vi "toCluster.vi"(3 "error in (no error)":errorcluster, 5 "PulseData in":refnum<class "PulseData.lvclass">) -> (0 "error out":errorcluster, 1 "Pulse Data Cluster":T1, 2 "PulseData out":refnum<class "PulseData.lvclass">)   [LabVIEW 2013, in "Controls Log Monitor.lvlib" / "PulseData.lvclass"]
uses:
  PulseData.lvclass
  PulseData.lvclass/PulseData.ctl
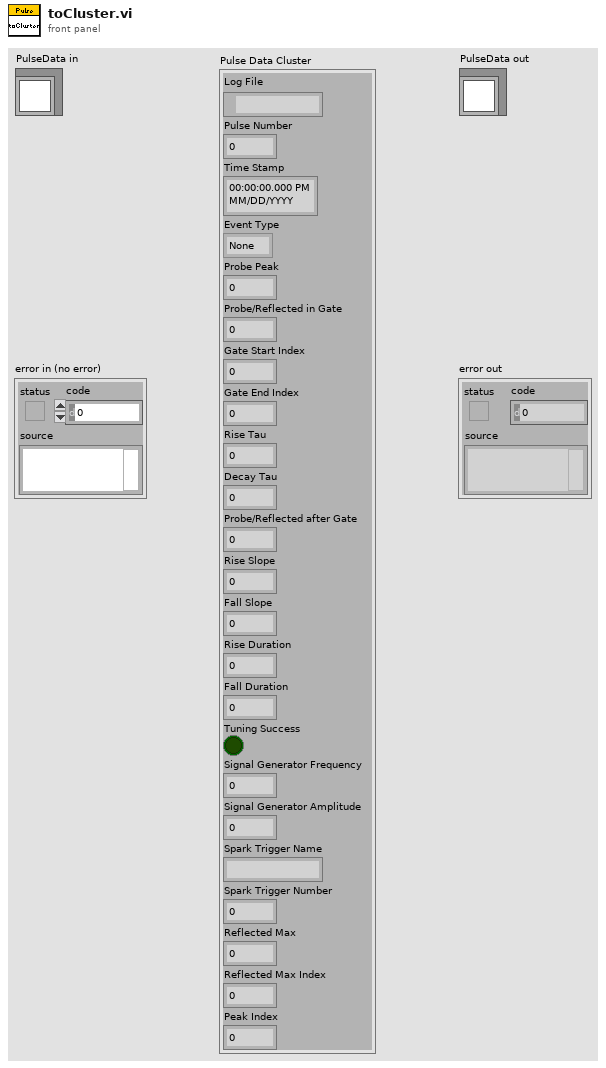
[diagram p1: front panel]
types:
  T1 = cluster{"Log File":path, "Pulse Number":u32, "Time Stamp":timestamp, "Event Type":enum16{"None", "Tune", "Periodic Capture", "Spark Trigger"}, "Probe Peak":dbl, "Probe/Reflected in Gate":dbl, "Gate Start Index":i32, "Gate End Index":i32, "Rise Tau":dbl, "Decay Tau":dbl, "Probe/Reflected after Gate":dbl, "Rise Slope":dbl, "Fall Slope":dbl, "Rise Duration":dbl, "Fall Duration":dbl, "Tuning Success":bool, "Signal Generator Frequency":dbl, "Signal Generator Amplitude":dbl, "Spark Trigger Name":string, "Spark Trigger Number":i32, "Reflected Max":dbl, "Reflected Max Index":i32, "Peak Index":i32}
  T2 = enum16{"None", "Tune", "Periodic Capture", "Spark Trigger"}
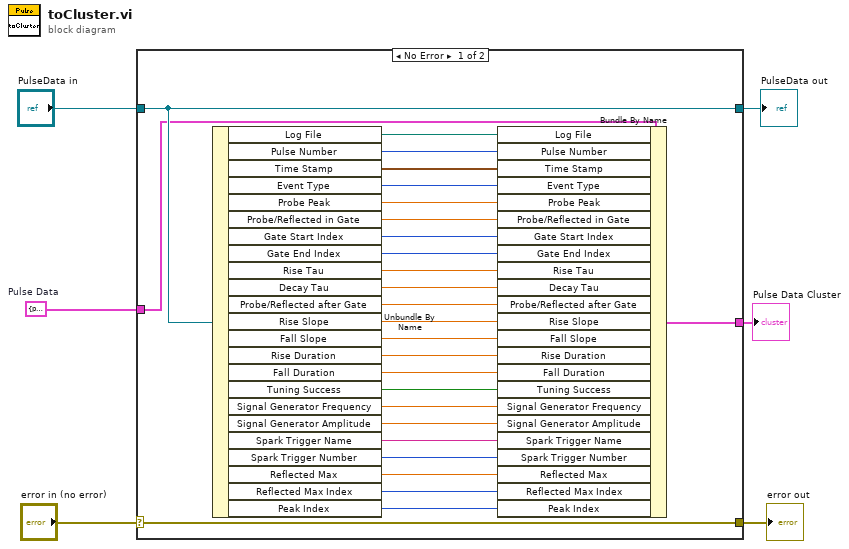
[diagram p0: block diagram]
diagram:
  w2 = T1 {"Log File"=path "", "Pulse Number"=0, "Time Stamp"=timestamp(0 s since 1904-01-01), "Event Type"=enum."None", "Probe Peak"=0.0, "Probe/Reflected in Gate"=0.0, "Gate Start Index"=0, "Gate End Index"=0, "Rise Tau"=0.0, "Decay Tau"=0.0, "Probe/Reflected after Gate"=0.0, "Rise Slope"=0.0, "Fall Slope"=0.0, "Rise Duration"=0.0, "Fall Duration"=0.0, "Tuning Success"=FALSE, "Signal Generator Frequency"=0.0, "Signal Generator Amplitude"=0.0, "Spark Trigger Name"="", "Spark Trigger Number"=0, "Reflected Max"=0.0, "Reflected Max Index"=0, "Peak Index"=0}  # Pulse Data
  n1 = case shown="No Error" "error in (no error)" {
    selector: "error in (no error)" -> [w33 w35]
    tunnel: [w33 w35] -> w5
    tunnel: [w32 w34] -> w3
    tunnel: "PulseData in" -> [w32 w34]
    tunnel: w2 -> [w31 _]
    tunnel: [w12 _] -> w1
    frame No Error {
      n2 = Unbundle By Name(w32) -> ("Log File"=w7:path, "Pulse Number"=w10:u32, "Time Stamp"=w11:timestamp, "Event Type"=w9:T2, "Probe Peak"=w30:dbl, "Probe/Reflected in Gate"=w29:dbl, "Gate Start Index"=w28:i32, "Gate End Index"=w27:i32, "Rise Tau"=w26:dbl, "Decay Tau"=w25:dbl, "Probe/Reflected after Gate"=w24:dbl, "Rise Slope"=w23:dbl, "Fall Slope"=w22:dbl, "Rise Duration"=w21:dbl, "Fall Duration"=w20:dbl, "Tuning Success"=w19:bool, "Signal Generator Frequency"=w18:dbl, "Signal Generator Amplitude"=w17:dbl, "Spark Trigger Name"=w16:string, "Spark Trigger Number"=w15:i32, "Reflected Max"=w14:dbl, "Reflected Max Index"=w13:i32, "Peak Index"=w8:i32)
      n3 = Bundle By Name(cluster=w31, "Log File"=w7, "Pulse Number"=w10, "Time Stamp"=w11, "Event Type"=w9, "Probe Peak"=w30, "Probe/Reflected in Gate"=w29, "Gate Start Index"=w28, "Gate End Index"=w27, "Rise Tau"=w26, "Decay Tau"=w25, "Probe/Reflected after Gate"=w24, "Rise Slope"=w23, "Fall Slope"=w22, "Rise Duration"=w21, "Fall Duration"=w20, "Tuning Success"=w19, "Signal Generator Frequency"=w18, "Signal Generator Amplitude"=w17, "Spark Trigger Name"=w16, "Spark Trigger Number"=w15, "Reflected Max"=w14, "Reflected Max Index"=w13, "Peak Index"=w8) -> (w12:T1)
    }
    frame Error {
    }
  }
  "error out" <- w5
  "PulseData out" <- w3
  "Pulse Data Cluster" <- w1
